vi "TripandIgnore.vi"(1 "Eval Period (s)":dbl, 2 "Signal In":bool) -> (0 "Tripped?":bool)   [LabVIEW 2016]
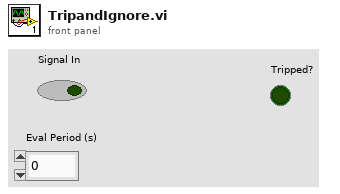
[diagram p1: front panel]
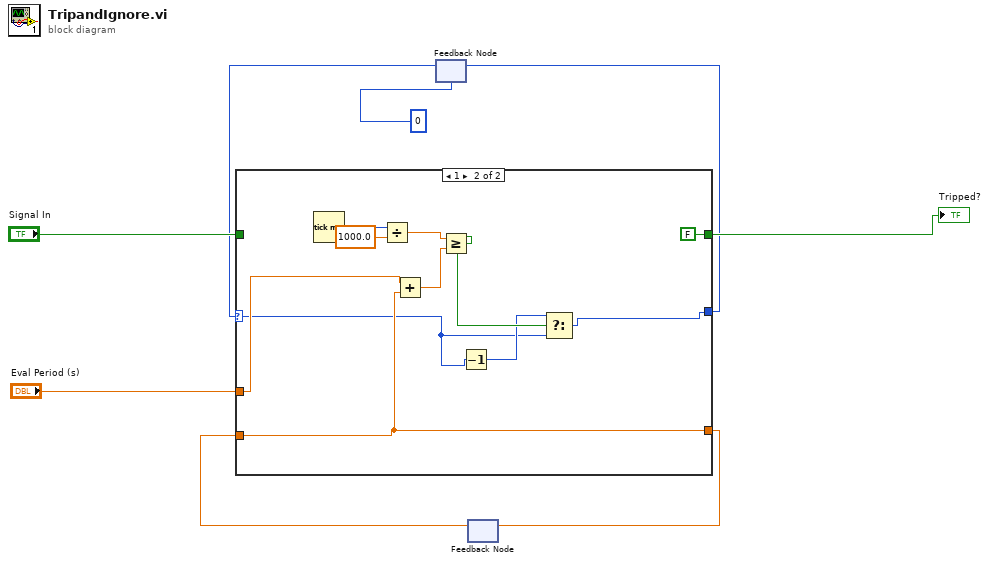
[diagram p0: block diagram]
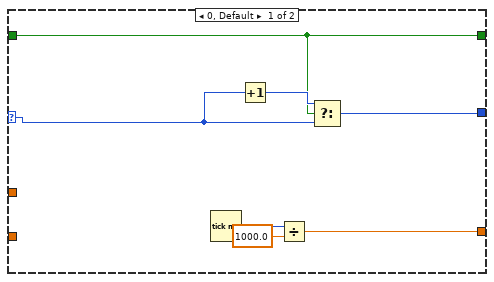
[diagram p2: hidden frame]
diagram:
  n1 = feedback #1(0) -> (w4:i32)
  n2 = feedback #2() -> (w1:dbl)  [unwired: 1 in]
  n3 = case shown="1" w4 {
    selector: w4 -> [w15 w16]
    tunnel: "Signal In" -> [w9 _]
    tunnel: [w9 FALSE ("Output")] -> w7
    tunnel: [w13 w19] -> w6
    tunnel: "Eval Period (s)" -> [_ w22]
    tunnel: [w10 w21] -> w2
    tunnel: w1 -> [_ w21]
    frame 0, Default {
      n4 = Tick Count (ms)() -> (millisecond timer value=w12:u32)
      n5 = Increment(x=w15) -> (x+1=w14:i32)
      n6 = Divide(x=w12, y=1000.0) -> (x/y=w10:dbl)
      n7 = Select(t=w14, s=w9, f=w15) -> (s? t:f=w13:i32)
    }
    frame 1 {
      n8 = Tick Count (ms)() -> (millisecond timer value=w26:u32)
      n9 = Divide(x=w26, y=1000.0) -> (x/y=w24:dbl)
      n10 = Add(x=w22, y=w21) -> (x+y=w23:dbl)
      n11 = Greater Or Equal?(x=w24, y=w23) -> (x >= y?=w20:bool)
      n12 = Decrement(x=w16) -> (x-1=w17:i32)
      n13 = Select(t=w17, s=w20, f=w16) -> (s? t:f=w19:i32)
    }
  }
  "Tripped?" <- w7
  n14 = feedback-in #1(w6) -> ()
  n15 = feedback-in #2(w2) -> ()
